vi "visionProcessing.vi"(7 "error in":errorcluster) -> (27 "error out":errorcluster)   [LabVIEW 2013]
uses:
  <vilib>/vision/NI_Vision_Development_Module.lvlib
panel:
  out "isFoundHorizontal":bool
  out "isFoundVertical":bool
  out "isFoundVertical":bool
  out "Image Out":T1(plugin-control)
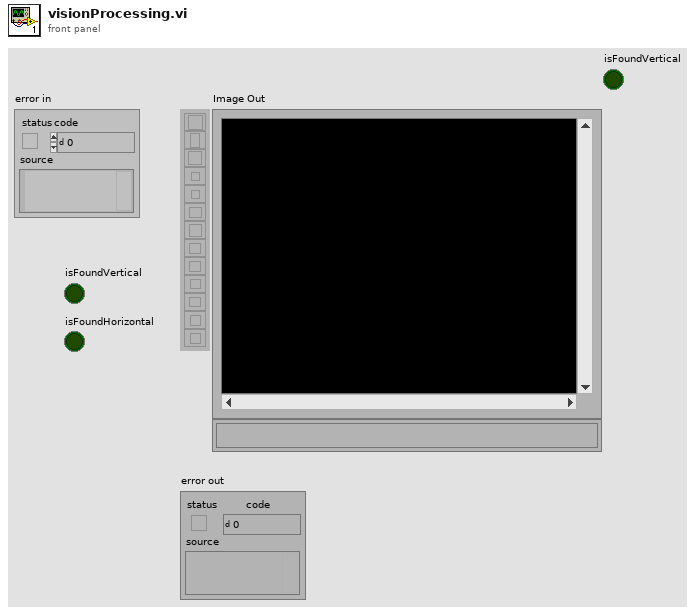
[diagram p1: front panel]
types:
  T1 = typedef "IMAQ Image.ctl" = refnum<image>
  T2 = typedef "Image Type" = u32
  T3 = cluster{"Global Rectangle":i32[], "Contours":cluster{"ID":enum32{"External", "Internal"}, "Type":u32, "Coordinates":i32[]}[]}
  T4 = cluster{"Position":cluster{"x":sgl, "y":sgl}, "Angle":sgl, "Scale":sgl, "Score":sgl, "Bounding Box":cluster{"x":sgl, "y":sgl}[]}[]
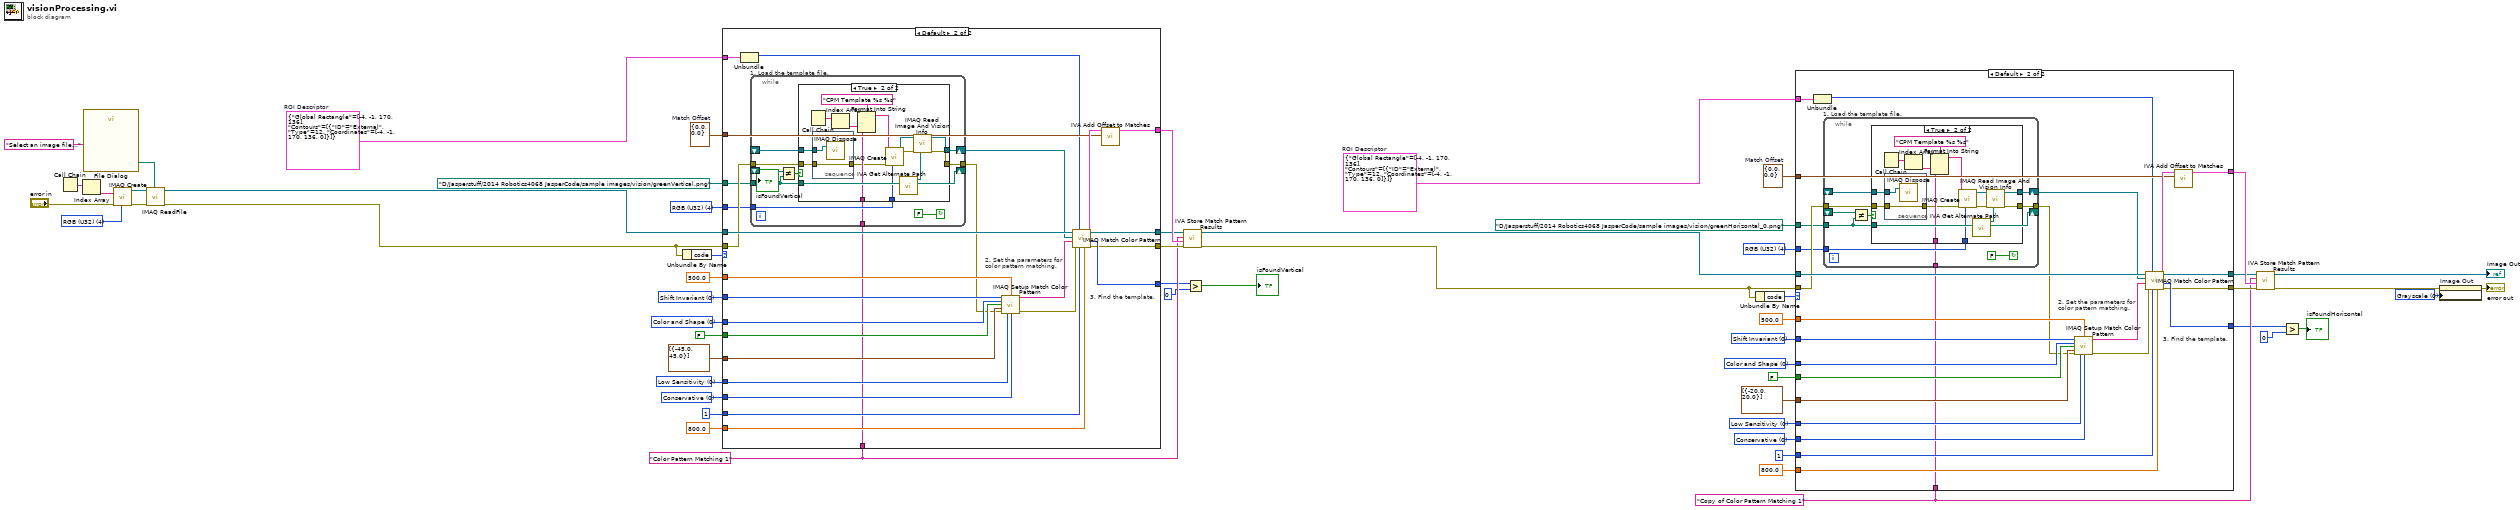
[diagram p0: block diagram]
diagram:
  w8 = u32 0 items=["Grayscale", "Binary", "Gradient", "Rainbow", "Temperature", "User Defined"] ("Palette")
  w10 = "Copy of Color Pattern Matching 1" ("Step Name")
  w20 = T2 4 items=["Grayscale (U8)", "Grayscale (I16)", "Grayscale (SGL)", "Complex (CSG)", "RGB (U32)", "HSL (U32)", "RGB (U64)"] ("Image Type")
  w18 = cluster{"X":sgl, "Y":sgl} {"X"=0.0, "Y"=0.0}  # Match Offset
  w23 = u32 0 items=["Conservative", "Balance", "Aggressive", "Very Aggressive"] ("Search Strategy")
  w24 = u32 0 items=["Low Sensitivity", "Medium Sensitivity", "High Sensitivity"] ("Color Sensitivity")
  w26 = u32 0 items=["Color and Shape", "Color", "Shape"] ("Match Feature Mode")
  w27 = u32 0 items=["Shift Invariant", "Rotation Invariant"] ("Match Mode")
  w17 = T3 {"Global Rectangle"=[-4, -1, 170, 136], "Contours"=[{"ID"=enum."External", "Type"=12, "Coordinates"=[-4, -1, 170, 136, 0]}]}  # ROI Descriptor
  w30 = "Color Pattern Matching 1" ("Step Name")
  w40 = T2 4 items=["Grayscale (U8)", "Grayscale (I16)", "Grayscale (SGL)", "Complex (CSG)", "RGB (U32)", "HSL (U32)", "RGB (U64)"] ("Image Type")
  w38 = cluster{"X":sgl, "Y":sgl} {"X"=0.0, "Y"=0.0}  # Match Offset
  w43 = u32 0 items=["Conservative", "Balance", "Aggressive", "Very Aggressive"] ("Search Strategy")
  w44 = u32 0 items=["Low Sensitivity", "Medium Sensitivity", "High Sensitivity"] ("Color Sensitivity")
  w46 = u32 0 items=["Color and Shape", "Color", "Shape"] ("Match Feature Mode")
  w47 = u32 0 items=["Shift Invariant", "Rotation Invariant"] ("Match Mode")
  w37 = T3 {"Global Rectangle"=[-4, -1, 170, 136], "Contours"=[{"ID"=enum."External", "Type"=12, "Coordinates"=[-4, -1, 170, 136, 0]}]}  # ROI Descriptor
  w50 = T2 4 items=["Grayscale (U8)", "Grayscale (I16)", "Grayscale (SGL)", "Complex (CSG)", "RGB (U32)", "HSL (U32)", "RGB (U64)", "Grayscale (U16)"] ("Image Type")
  n1 = Call Chain() -> (call chain=w54:string[])
  n2 = Index Array(array=w54) -> (element=w53:string)  [unwired: 1 in]
  n3 = call "File Dialog"("prompt"="Select an image file...") -> ("selected path"=w51:path)  [unwired: 6 in, 8 out]
  n4 = call "IMAQ Create"("Image Name"=w53, "Image Type"=w50, "error in (no error)"="error in") -> ("New Image"=w57:T1, "error out"=w56:errorcluster)  [unwired: 1 in, 1 out]
  n5 = call "IMAQ ReadFile"("File Path"=w51, "error in (no error)"=w56, "Image"=w57) -> ("error out"=w58:errorcluster, "Image Out"=w36:T1)  [unwired: 2 in, 5 out]
  n6 = Unbundle By Name(w58) -> ("code"=w35:i32)
  n7 = case shown="Default" w35 {
    tunnel: 1 ("Number of Matches Requested") -> [_ w84]
    tunnel: sgl 800.0 ("Minimum Match Score") -> [_ w83]
    tunnel: [_ w82] -> w6
    tunnel: w47 -> [_ w81]
    tunnel: w46 -> [_ w80]
    tunnel: FALSE ("Subpixel Accuracy") -> [_ w79]
    tunnel: w44 -> [_ w78]
    tunnel: w43 -> [_ w77]
    tunnel: sgl 500.0 ("Color Score Weight") -> [_ w76]
    tunnel: path "D:/Jasperstuff/2014 Robotics4068 JasperCode/sample images/vision/greenVertical.png" ("File Path") -> [_ w65]
    tunnel: w40 -> [_ w61]
    tunnel: w58 -> [_ w66]
    tunnel: cluster{sgl, sgl}[] [{-45.0, 45.0}] ("Rotation Angle Ranges (degrees)") -> [_ w73]
    tunnel: w38 -> [_ w71]
    tunnel: w37 -> [_ w70]
    tunnel: [_ w62] -> w32
    tunnel: w36 -> [w59 w67]
    tunnel: [w59 w67] -> w31
    tunnel: [_ w68] -> w34
    tunnel: w30 -> [_ w60]
    frame -1074396199, -1074396198 {
      # "Discard Coordinate System Error"
    }
    frame Default {
      # "2. Set the parameters for\ncolor pattern matching."
      # "3. Find the template."
      n8 = Unbundle(w70) -> ("Global Rectangle"=w69:i32[])  [unwired: 1 out]
      n9 = while "1. Load the template file." {
        shift-right: [w94] -> w64
        shift-left: _ -> [w93]
        tunnel: [w91] -> w63
        tunnel: w66 -> [w90]
        tunnel: w65 -> [w85]
        tunnel: w61 -> [w89]
        tunnel: w60 -> [w88]
        shift-right: [w85] -> _
        shift-left: _ -> [w87]
        stop <- FALSE continue-if-true
        n10 = Not Equal?(x=w87, y=w85) -> (x != y?=w86:bool)
        n11 = case shown="True" w86 {
          tunnel: [w96 w109] -> w94
          tunnel: w93 -> [w96 w101]
          tunnel: [w95 w106] -> w91
          tunnel: w90 -> [w95 w100]
          tunnel: w85 -> [_ w98]
          tunnel: w89 -> [_ w105]
          tunnel: w88 -> [_ w102]
          frame False {
          }
          frame True {
            n12 = Call Chain() -> (call chain=w104:string[])
            n13 = stacked-sequence {
              tunnel: w101 -> [w113]
              tunnel: w100 -> [w112]
              tunnel: [w112] -> w99
              frame #0 {
                n14 = call "IMAQ Dispose"("Image"=w113) -> ()  [unwired: 2 in, 4 out]
              }
            }
            n15 = Index Array(array=w104) -> (element=w103:string)  [unwired: 1 in]
            n16 = Format Into String(format string="CPM Template %s %s" ("Image Name"), w103, w102) -> (resulting string=w111:string)  [unwired: 2 in, 1 out]
            n17 = call "IMAQ Create"("Image Name"=w111, "Image Type"=w105, "error in (no error)"=w99) -> ("New Image"=w108:T1, "error out"=w107:errorcluster)  [unwired: 1 in, 1 out]
            n18 = call <vilib>:"IVA Get Alternate Path.vi"("Path In"=w98) -> ("Path Out"=w97:path)  [unwired: 10 out]
            n19 = call "IMAQ Read Image And Vision Info"("File Path"=w97, "error in (no error)"=w107, "Image"=w108) -> ("error out"=w106:errorcluster, "Image Out"=w109:T1)  [unwired: 1 in, 6 out]
          }
        }
      }
      n20 = call "IMAQ Setup Match Color Pattern"("Match Mode"=w81, "Color Score Weight"=w76, "Match Feature Mode"=w80, "Subpixel Accuracy"=w79, "Rotation Angle Ranges (degrees)"=w73, "error in (no error)"=w63, "Color Sensitivity"=w78, "Search Strategy"=w77) -> ("Match Color Pattern Setup Data"=w75:string, "error out"=w74:errorcluster)  [unwired: 1 in, 5 out]
      n21 = call "IMAQ Match Color Pattern"("Minimum Match Score"=w83, "Number of Matches Requested"=w84, "Optional Rectangle"=w69, "error in (no error)"=w74, "Match Color Pattern Setup Data"=w75, "Template Image"=w64, "Image"=w67) -> ("error out"=w62:errorcluster, "Number of Matches"=w82:i32, "Matches"=w72:T4)  [unwired: 2 out]
      n22 = call <vilib>:"IVA Add Offset to Matches.vi"("Match Offset"=w71, "Matches in"=w72) -> ("Matches out"=w68:T4)  [unwired: 9 out]
    }
  }
  n23 = call <vilib>:"IVA Store Match Pattern Results.vi"("error in (no error)"=w32, "Matches"=w34, "Step Name"=w30, "Image in"=w31) -> ("error out"=w33:errorcluster, "Image dup"=w16:T1)  [unwired: 6 out]
  n24 = Greater?(x=w6, y=0) -> (0:→"isFoundVertical":bool)
  n25 = Unbundle By Name(w33) -> ("code"=w15:i32)
  n26 = case shown="Default" w15 {
    tunnel: 1 ("Number of Matches Requested") -> [_ w139]
    tunnel: sgl 800.0 ("Minimum Match Score") -> [_ w138]
    tunnel: [_ w137] -> w2
    tunnel: w27 -> [_ w136]
    tunnel: w26 -> [_ w135]
    tunnel: FALSE ("Subpixel Accuracy") -> [_ w134]
    tunnel: w24 -> [_ w133]
    tunnel: w23 -> [_ w132]
    tunnel: sgl 500.0 ("Color Score Weight") -> [_ w131]
    tunnel: path "D:/Jasperstuff/2014 Robotics4068 JasperCode/sample images/vision/greenHorizontal_0.png" ("File Path") -> [_ w120]
    tunnel: w20 -> [_ w116]
    tunnel: w33 -> [_ w121]
    tunnel: cluster{sgl, sgl}[] [{-20.0, 20.0}] ("Rotation Angle Ranges (degrees)") -> [_ w128]
    tunnel: w18 -> [_ w126]
    tunnel: w17 -> [_ w125]
    tunnel: [_ w117] -> w12
    tunnel: w16 -> [w114 w122]
    tunnel: [w114 w122] -> w11
    tunnel: [_ w123] -> w14
    tunnel: w10 -> [_ w115]
    frame -1074396199, -1074396198 {
      # "Discard Coordinate System Error"
    }
    frame Default {
      # "2. Set the parameters for\ncolor pattern matching."
      # "3. Find the template."
      n27 = Unbundle(w125) -> ("Global Rectangle"=w124:i32[])  [unwired: 1 out]
      n28 = while "1. Load the template file." {
        shift-right: [w149] -> w119
        shift-left: _ -> [w148]
        tunnel: [w146] -> w118
        tunnel: w121 -> [w145]
        tunnel: w120 -> [w140]
        tunnel: w116 -> [w144]
        tunnel: w115 -> [w143]
        shift-right: [w140] -> _
        shift-left: _ -> [w142]
        stop <- FALSE continue-if-true
        n29 = Not Equal?(x=w142, y=w140) -> (x != y?=w141:bool)
        n30 = case shown="True" w141 {
          tunnel: [w151 w164] -> w149
          tunnel: w148 -> [w151 w156]
          tunnel: [w150 w161] -> w146
          tunnel: w145 -> [w150 w155]
          tunnel: w140 -> [_ w153]
          tunnel: w144 -> [_ w160]
          tunnel: w143 -> [_ w157]
          frame False {
          }
          frame True {
            n31 = Call Chain() -> (call chain=w159:string[])
            n32 = stacked-sequence {
              tunnel: w156 -> [w168]
              tunnel: w155 -> [w167]
              tunnel: [w167] -> w154
              frame #0 {
                n33 = call "IMAQ Dispose"("Image"=w168) -> ()  [unwired: 2 in, 4 out]
              }
            }
            n34 = Index Array(array=w159) -> (element=w158:string)  [unwired: 1 in]
            n35 = Format Into String(format string="CPM Template %s %s" ("Image Name"), w158, w157) -> (resulting string=w166:string)  [unwired: 2 in, 1 out]
            n36 = call "IMAQ Create"("Image Name"=w166, "Image Type"=w160, "error in (no error)"=w154) -> ("New Image"=w163:T1, "error out"=w162:errorcluster)  [unwired: 1 in, 1 out]
            n37 = call <vilib>:"IVA Get Alternate Path.vi"("Path In"=w153) -> ("Path Out"=w152:path)  [unwired: 10 out]
            n38 = call "IMAQ Read Image And Vision Info"("File Path"=w152, "error in (no error)"=w162, "Image"=w163) -> ("error out"=w161:errorcluster, "Image Out"=w164:T1)  [unwired: 1 in, 6 out]
          }
        }
      }
      n39 = call "IMAQ Setup Match Color Pattern"("Match Mode"=w136, "Color Score Weight"=w131, "Match Feature Mode"=w135, "Subpixel Accuracy"=w134, "Rotation Angle Ranges (degrees)"=w128, "error in (no error)"=w118, "Color Sensitivity"=w133, "Search Strategy"=w132) -> ("Match Color Pattern Setup Data"=w130:string, "error out"=w129:errorcluster)  [unwired: 1 in, 5 out]
      n40 = call "IMAQ Match Color Pattern"("Minimum Match Score"=w138, "Number of Matches Requested"=w139, "Optional Rectangle"=w124, "error in (no error)"=w129, "Match Color Pattern Setup Data"=w130, "Template Image"=w119, "Image"=w122) -> ("error out"=w117:errorcluster, "Number of Matches"=w137:i32, "Matches"=w127:T4)  [unwired: 2 out]
      n41 = call <vilib>:"IVA Add Offset to Matches.vi"("Match Offset"=w126, "Matches in"=w127) -> ("Matches out"=w123:T4)  [unwired: 9 out]
    }
  }
  n42 = call <vilib>:"IVA Store Match Pattern Results.vi"("error in (no error)"=w12, "Matches"=w14, "Step Name"=w10, "Image in"=w11) -> ("error out"=w13:errorcluster, "Image dup"=→"Image Out":T1)  [unwired: 6 out]
  n43 = Greater?(x=w2, y=0) -> (0:→"isFoundHorizontal":bool)
  n44 = property on="Image Out" class="ImageControl"(error in=w13, "Palette:Palette Type"=w8) -> (error out=→"error out":errorcluster)  [unwired: 1 in, 1 out]
